vi "ma_SML Spectrum Peak Search (advanced).vi"(4 "# expected peaks":i32=-1, 6 "threshold":dbl format="%.2f", 7 "peaks near frequencies":T1={"Frequencies"=[], "Tolerance (Hz)"=100.0} {"Tolerance (Hz)" format="%_4p"; "Frequencies" format="%_4p"}, 8 "error in (no error)":errorcluster, 9 "peak search mode":u16(ring) items=["Threshold", "Highest N Peaks", "Peaks Near Frequencies"], 10 "spectral info":T2 {"window" items=["Rectangle"=0, "Hanning"=1, "Hamming"=2, "Blackman-Harris"=3, "Exact Blackman"=4, "Blackman"=5, "Flat Top"=6, "4 Term B-Harris "=7, "7 Term B-Harris"=8, "Low Sidelobe"=9, "Blackman Nuttall"=11, "Triangle"=30, "Bartlett-Hanning"=31, "Bohman"=32, "Parzen"=33, "Welch"=34, "Kaiser"=60, "Dolph-Chebyshev"=61, "Gaussian"=62]}, 11 "spectrum":T3={"f0"=1.0, "df"=1.0, "spectrum"=[]} {"spectrum" format="%.2f"; "df" format="%.2f"; "f0" format="%.2f"}) -> (0 "error out":errorcluster, 2 "# peaks":i32, 3 "peaks":cluster{"frequency":dbl, "value":dbl}[](array[cluster]) {"value" format="%.2f"; "frequency" format="%.2f"})   [LabVIEW 2020, in "NI_MAPro.lvlib"]
uses:
  NI_MAPro.lvlib
  ma_sml_Spectrum Cluster (real).ctl
  ma_sml_Spectral Info.ctl
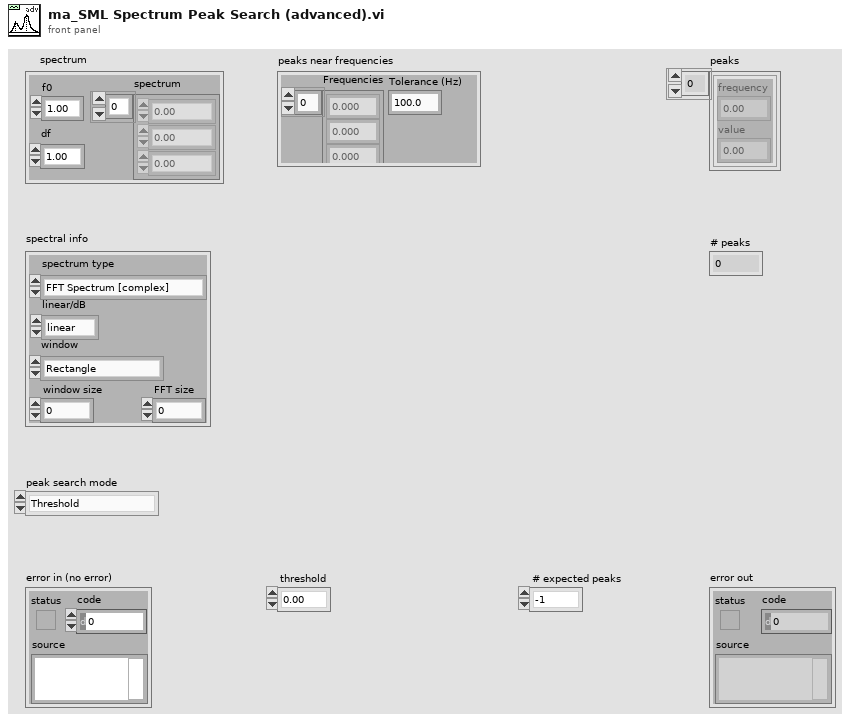
[diagram p1: front panel]
types:
  T1 = cluster{"Frequencies":dbl[], "Tolerance (Hz)":dbl}
  T2 = typedef "NI_MAPro.lvlib/ma_sml_Spectral Info.ctl" = cluster{"spectrum type":enum16{"FFT Spectrum [complex]", "Amplitude [Magnitude]", "Power [Magnitude^2]", "Cross Spectrum [complex]", "Frequency Response [Complex]"}, "linear/dB":enum16{"linear", "dB"}, "window":u16, "window size":i32, "FFT size":i32}
  T3 = typedef "NI_MAPro.lvlib/ma_sml_Spectrum Cluster (real).ctl" = cluster{"f0":dbl, "df":dbl, "spectrum":dbl[]}
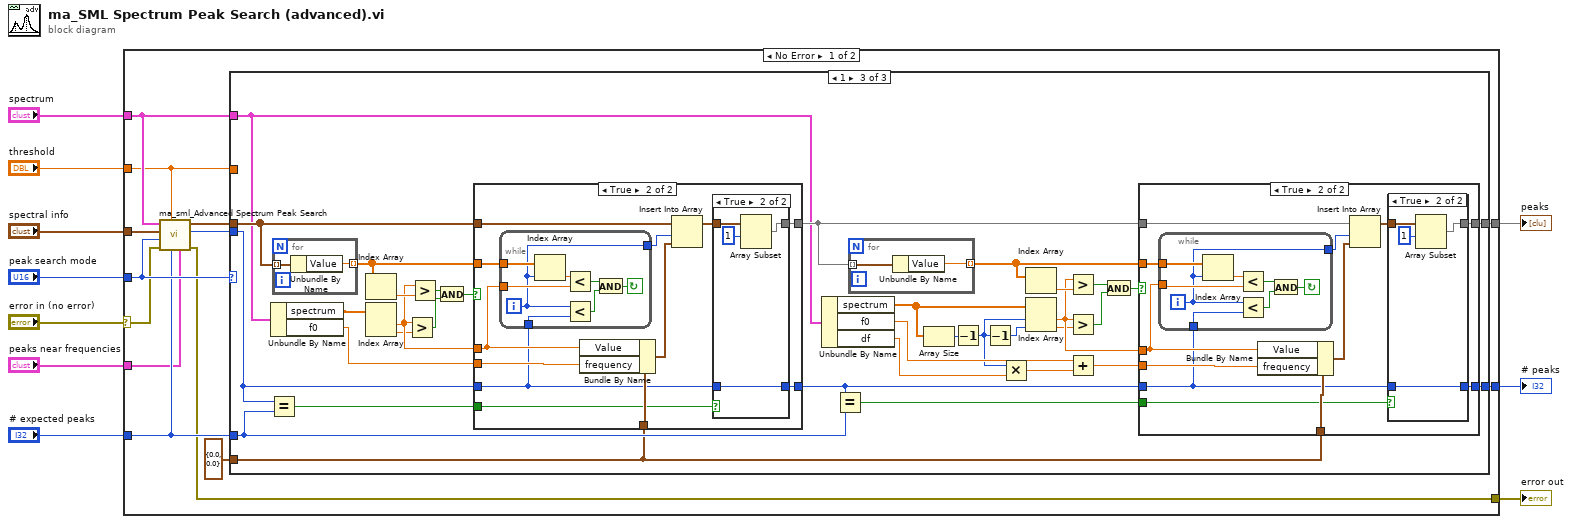
[diagram p0: block diagram]
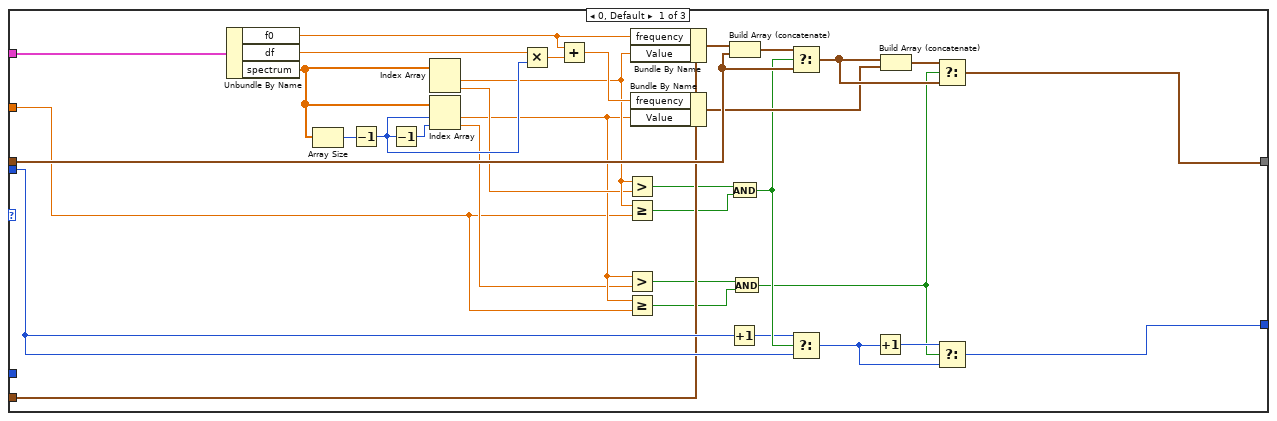
[diagram p2: hidden frame]
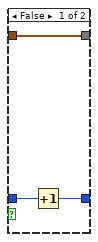
[diagram p5: hidden frame]
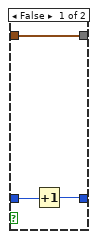
[diagram p7: hidden frame]
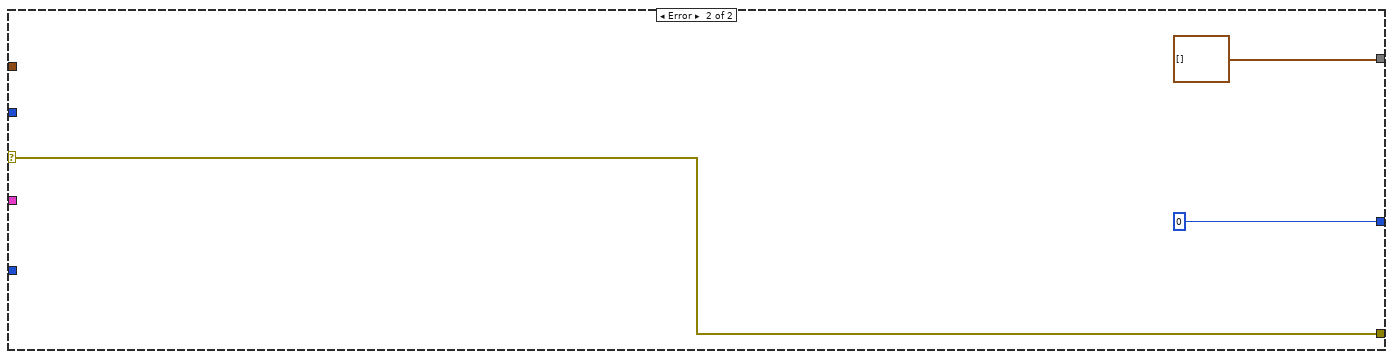
[diagram p8: hidden frame]
diagram:
  n1 = case shown="No Error" "error in (no error)" {
    selector: "error in (no error)" -> [w16 w158]
    tunnel: "spectrum" -> [w21 _]
    tunnel: "spectral info" -> [w20 _]
    tunnel: [w23 cluster{"frequency":dbl, "Value":dbl}[] [] ("peaks")] -> w8
    tunnel: [w22 0 ("# of peaks")] -> w7
    tunnel: [w13 w158] -> w6
    tunnel: "threshold" -> [w17 _]
    tunnel: "# expected peaks" -> [w18 _]
    tunnel: "peak search mode" -> [w19 _]
    tunnel: "peaks near frequencies" -> [w11 _]
    frame No Error {
      n2 = call "ma_sml_Advanced Spectrum Peak Search.vi"("peaks near frequencies"=w11, "highest n peaks"=w18, "threshold"=w17, "error in (no error)"=w16, "peak search mode"=w19, "spectral info"=w20, "spectrum"=w21) -> ("error out"=w13:errorcluster, "# of peaks"=w14:i32, "peaks"=w15:cluster{"frequency":dbl, "Value":dbl}[])  [unwired: 2 in]
      n3 = case shown="1" w19 {
        tunnel: w21 -> [w56 _ w87]
        tunnel: w15 -> [w51 w58 w92]
        tunnel: w17 -> [w27 _ _]
        tunnel: [w40 w58 w86] -> w23
        tunnel: [w39 w57 w85] -> w22
        tunnel: w14 -> [w38 w57 w91]
        tunnel: w18 -> [_ _ w89]
        tunnel: cluster{"frequency":dbl, "Value":dbl} {"frequency"=0.0, "Value"=0.0} -> [w36 _ w84]
        frame 0, Default {
          n4 = Unbundle By Name(w56) -> ("f0"=w48:dbl, "df"=w37:dbl, "spectrum"=w55:dbl[])
          n5 = Array Size(array=w55) -> (size(s)=w50:i32)
          n6 = Decrement(x=w50) -> (x-1=w35:i32)
          n7 = Decrement(x=w35) -> (x-1=w34:i32)
          n8 = Index Array(array=w55) -> (element #1=w33:dbl, element #2=w32:dbl)  [unwired: 2 in]
          n9 = Index Array(array=w55, index #1=w35, index #2=w34) -> (element #1=w31:dbl, element #2=w30:dbl)
          n10 = Multiply(x=w37, y=w35) -> (x*y=w49:dbl)
          n11 = Add(x=w48, y=w49) -> (x+y=w47:dbl)
          n12 = Greater?(x=w33, y=w32) -> (0:w29:bool)
          n13 = Greater Or Equal?(x=w33, y=w27) -> (x >= y?=w28:bool)
          n14 = Greater?(x=w31, y=w30) -> (0:w26:bool)
          n15 = Greater Or Equal?(x=w31, y=w27) -> (x >= y?=w25:bool)
          n16 = Bundle By Name(cluster=w36, "frequency"=w48, "Value"=w33) -> (w54:cluster{"frequency":dbl, "Value":dbl})
          n17 = Bundle By Name(cluster=w36, "frequency"=w47, "Value"=w31) -> (w45:cluster{"frequency":dbl, "Value":dbl})
          n18 = Increment(x=w38) -> (x+1=w43:i32)
          n19 = Build Array (concatenate)(w54, w51) -> (w53:cluster{"frequency":dbl, "Value":dbl}[])
          n20 = And(x=w29, y=w28) -> (x .and. y?=w44:bool)
          n21 = And(x=w26, y=w25) -> (x .and. y?=w24:bool)
          n22 = Select(t=w53, s=w44, f=w51) -> (s? t:f=w46:cluster{"frequency":dbl, "Value":dbl}[])
          n23 = Select(t=w43, s=w44, f=w38) -> (s? t:f=w42:i32)
          n24 = Increment(x=w42) -> (x+1=w41:i32)
          n25 = Build Array (concatenate)(w46, w45) -> (w52:cluster{"frequency":dbl, "Value":dbl}[])
          n26 = Select(t=w52, s=w24, f=w46) -> (s? t:f=w40:cluster{"frequency":dbl, "Value":dbl}[])
          n27 = Select(t=w41, s=w24, f=w42) -> (s? t:f=w39:i32)
        }
        frame 2 {
        }
        frame 1 {
          n28 = Equal?(x=w91, y=w89) -> (x = y?=w93:bool)
          n29 = Unbundle By Name(w87) -> ("spectrum"=w77:dbl[], "f0"=w81:dbl)
          n30 = for {
            tunnel: w92 -> [w126] mode=indexing
            tunnel: [w125] -> w82 mode=indexing
            n31 = Unbundle By Name(w126) -> ("Value"=w125:dbl)
          }
          n32 = Index Array(array=w82) -> (element=w83:dbl)  [unwired: 1 in]
          n33 = Index Array(array=w77) -> (element #1=w80:dbl, element #2=w79:dbl)  [unwired: 2 in]
          n34 = Greater?(x=w80, y=w79) -> (0:w76:bool)
          n35 = Greater?(x=w80, y=w83) -> (0:w75:bool)
          n36 = And(x=w75, y=w76) -> (x .and. y?=w78:bool)
          n37 = case shown="True" w78 {
            tunnel: w82 -> [_ w139]
            tunnel: w81 -> [_ w132]
            tunnel: w80 -> [_ w138]
            tunnel: w92 -> [w128 w136]
            tunnel: [w128 w134] -> w90
            tunnel: w91 -> [w127 w130]
            tunnel: [w127 w129] -> w88
            tunnel: w84 -> [_ w133]
            tunnel: w93 -> [_ w131]
            frame False {
            }
            frame True {
              n38 = while {
                tunnel: w139 -> [w155]
                tunnel: w138 -> [w153]
                tunnel: [w151] -> w140
                tunnel: w130 -> [w150]
                i -> [w151]
                stop <- w148 continue-if-true
                n39 = Index Array(array=w155, index=w151) -> (element=w154:dbl)
                n40 = Less?(x=w154, y=w153) -> (x < y?=w152:bool)
                n41 = Less?(x=w151, y=w150) -> (x < y?=w149:bool)
                n42 = And(x=w152, y=w149) -> (x .and. y?=w148:bool)
              }
              n43 = Bundle By Name(cluster=w133, "Value"=w138, "frequency"=w132) -> (w137:cluster{"frequency":dbl, "Value":dbl})
              n44 = Insert Into Array(array=w136, index=w140, new element=w137) -> (w135:cluster{"frequency":dbl, "Value":dbl}[])
              n45 = case shown="True" w131 {
                tunnel: w135 -> [w143 w146]
                tunnel: [w143 w145] -> w134
                tunnel: w130 -> [w141 w144]
                tunnel: [w142 w144] -> w129
                frame False {
                  n46 = Increment(x=w141) -> (x+1=w142:i32)
                }
                frame True {
                  n47 = Array Subset(array=w146, index=1) -> (w145:cluster{"frequency":dbl, "Value":dbl}[])  [unwired: 1 in]
                }
              }
            }
          }
          n48 = Unbundle By Name(w87) -> ("spectrum"=w67:dbl[], "f0"=w71:dbl, "df"=w72:dbl)
          n49 = Equal?(x=w88, y=w89) -> (x = y?=w59:bool)
          n50 = for {
            tunnel: w90 -> [w95] mode=indexing
            tunnel: [w94] -> w73 mode=indexing
            n51 = Unbundle By Name(w95) -> ("Value"=w94:dbl)
          }
          n52 = Array Size(array=w67) -> (size(s)=w69:i32)
          n53 = Decrement(x=w69) -> (x-1=w66:i32)
          n54 = Decrement(x=w66) -> (x-1=w65:i32)
          n55 = Multiply(x=w66, y=w72) -> (x*y=w70:dbl)
          n56 = Index Array(array=w73) -> (element=w74:dbl)  [unwired: 1 in]
          n57 = Index Array(array=w67, index #1=w66, index #2=w65) -> (element #1=w64:dbl, element #2=w63:dbl)
          n58 = Greater?(x=w64, y=w74) -> (0:w61:bool)
          n59 = Greater?(x=w64, y=w63) -> (0:w62:bool)
          n60 = Add(x=w71, y=w70) -> (x+y=w68:dbl)
          n61 = And(x=w61, y=w62) -> (x .and. y?=w60:bool)
          n62 = case shown="True" w60 {
            tunnel: w73 -> [_ w108]
            tunnel: w68 -> [_ w101]
            tunnel: w64 -> [_ w107]
            tunnel: w90 -> [w97 w105]
            tunnel: [w97 w103] -> w86
            tunnel: w88 -> [w96 w99]
            tunnel: [w96 w98] -> w85
            tunnel: w84 -> [_ w102]
            tunnel: w59 -> [_ w100]
            frame False {
            }
            frame True {
              n63 = while {
                tunnel: w108 -> [w124]
                tunnel: w107 -> [w122]
                tunnel: [w121] -> w109
                tunnel: w99 -> [w120]
                i -> [w121]
                stop <- w117 continue-if-true
                n64 = Index Array(array=w124, index=w121) -> (element=w123:dbl)
                n65 = Less?(x=w123, y=w122) -> (x < y?=w119:bool)
                n66 = Less?(x=w121, y=w120) -> (x < y?=w118:bool)
                n67 = And(x=w119, y=w118) -> (x .and. y?=w117:bool)
              }
              n68 = Bundle By Name(cluster=w102, "Value"=w107, "frequency"=w101) -> (w106:cluster{"frequency":dbl, "Value":dbl})
              n69 = Insert Into Array(array=w105, index=w109, new element=w106) -> (w104:cluster{"frequency":dbl, "Value":dbl}[])
              n70 = case shown="True" w100 {
                tunnel: w104 -> [w110 w115]
                tunnel: [w110 w114] -> w103
                tunnel: w99 -> [w111 w113]
                tunnel: [w112 w113] -> w98
                frame False {
                  n71 = Increment(x=w111) -> (x+1=w112:i32)
                }
                frame True {
                  n72 = Array Subset(array=w115, index=1) -> (w114:cluster{"frequency":dbl, "Value":dbl}[])  [unwired: 1 in]
                }
              }
            }
          }
        }
      }
    }
    frame Error {
    }
  }
  "peaks" <- w8
  "error out" <- w6
  "# peaks" <- w7
